vi "Prepare.vi"(8 "error in (no error)":errorcluster, 9 "Wavefom Sequence":T4, 10 "TDMS Name Mapping":T3, 11 "Resource Settings":T2={"FGEN Resource"="", "DAQmx Resource"="", "TDMS File Path"=path "", "Scope Resource"="", "Scope Config File Path"=path "", "Reference Position"=50.0} {"Reference Position" format="%#_g%"}) -> (0 "error out":errorcluster, 3 "Panel State Data Out":T1)   [LabVIEW 2025]
uses:
  Typedef/Test Panel State Data.ctl
  a73cb824-e8e3-43f7-ba20-95578727caf9.vi
  51479c3b-831f-4f08-87c6-485a7376d69e.vi
  Typedef/TDMS Name Mapping.ctl
  Typedef/Resource Settings.ctl
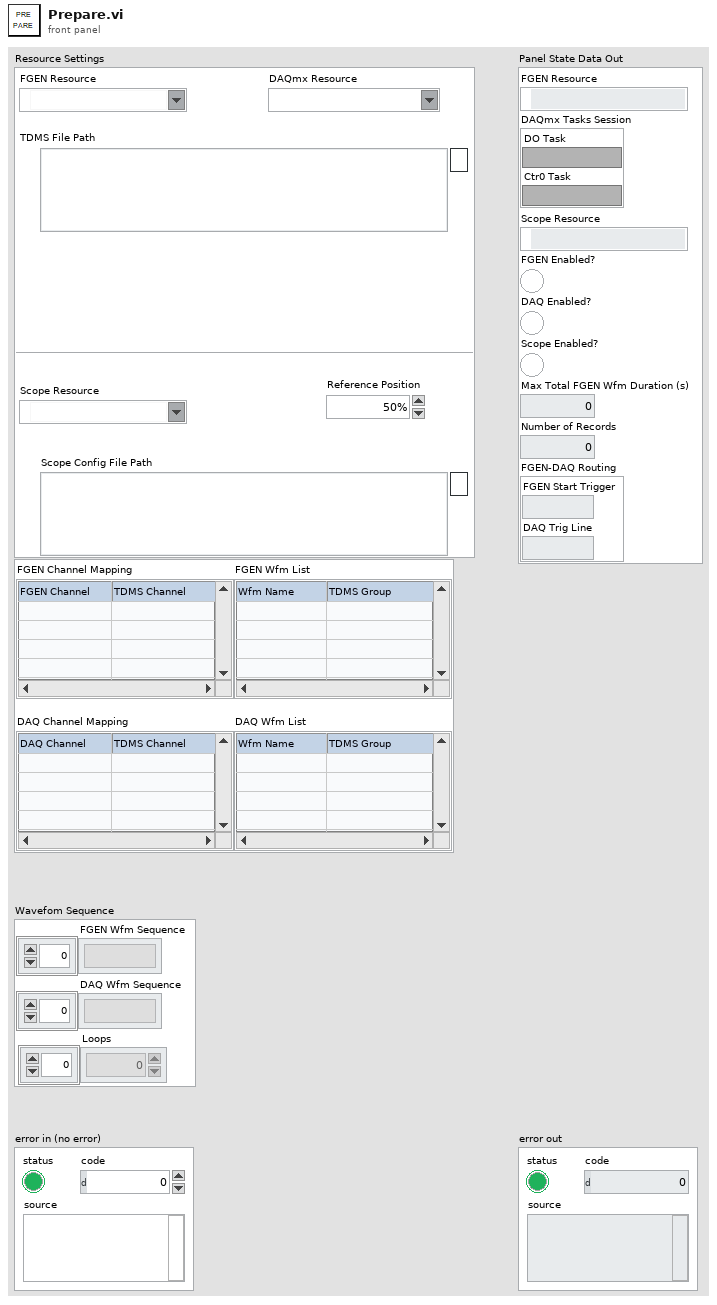
[diagram p1: front panel]
types:
  T1 = typedef "Test Panel State Data.ctl" = cluster{"FGEN Resource":refnum<k15>, "DAQmx Tasks Session":cluster{"DO Task":refnum<k21>, "Ctr0 Task":refnum<k21>}, "Scope Resource":refnum<k15>, "FGEN Enabled?":bool, "DAQ Enabled?":bool, "Scope Enabled?":bool, "Max Total FGEN Wfm Duration (s)":dbl, "Number of Records":i32, "FGEN-DAQ Routing":cluster{"FGEN Start Trigger":string, "DAQ Trig Line":string}}
  T2 = typedef "Resource Settings.ctl" = cluster{"FGEN Resource":refnum<k15>, "DAQmx Resource":tag, "TDMS File Path":path, "Scope Resource":refnum<k15>, "Scope Config File Path":path, "Reference Position":dbl}
  T3 = typedef "TDMS Name Mapping.ctl" = cluster{"FGEN Channel Mapping":string[][], "DAQ Channel Mapping":string[][], "FGEN Wfm List":string[][], "DAQ Wfm List":string[][]}
  T4 = cluster{"FGEN Wfm Sequence":string[], "DAQ Wfm Sequence":string[], "Loops":i32[]}
  T5 = cluster{"DAQ Channels":string[], "Sample Rate":dbl, "DAQ Wfm Map":map{string, digitalwaveform}, "DAQ Wfm Sequence":string[], "Loops":i32[]}
  T6 = cluster{"FGEN Channels":string[], "Sample Rate":dbl, "FGEN Wfm Map":map{string, waveform(dbl)[]}, "FGEN Wfm Sequence":string[], "Loops":i32[], "Gain Per Channel":dbl[]}
  T7 = cluster{"DO Task":refnum<k21>, "Ctr0 Task":refnum<k21>}
  T8 = cluster{"Scope Config File Path":path, "Reference Position":dbl, "Numeric":i32}
  T9 = cluster{"FGEN Start Trigger":string, "DAQ Trig Line":string}
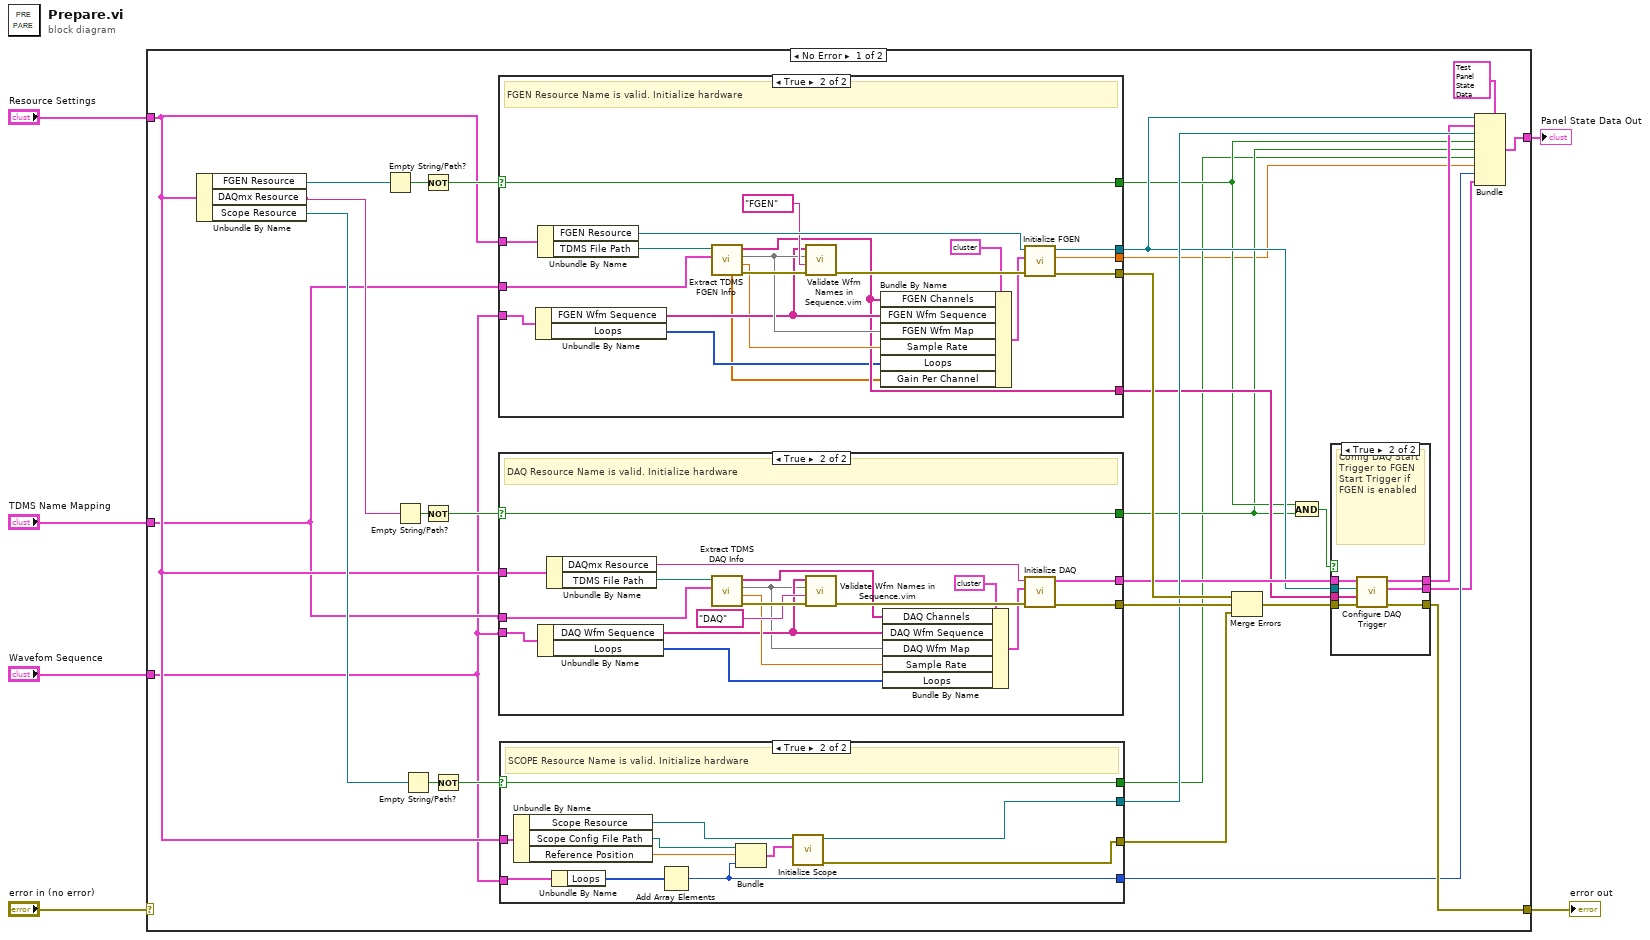
[diagram p0: block diagram]
diagram:
  n1 = case shown="No Error" "error in (no error)" {
    selector: "error in (no error)" -> [_ w99]
    tunnel: "Resource Settings" -> [w24 _]
    tunnel: "TDMS Name Mapping" -> [w21 _]
    tunnel: "Wavefom Sequence" -> [w20 _]
    tunnel: [w14 w99] -> w6
    tunnel: [w37 _] -> w1
    frame No Error {
      n2 = Unbundle By Name(w24) -> ("FGEN Resource"=w36:refnum<k15>, "DAQmx Resource"=w35:tag, "Scope Resource"=w34:refnum<k15>)
      n3 = Empty String/Path?(string/path=w36) -> (empty?=w33:bool)
      n4 = Empty String/Path?(string/path=w35) -> (empty?=w30:bool)
      n5 = Empty String/Path?(string/path=w34) -> (empty?=w26:bool)
      n6 = Not(x=w33) -> (.not. x?=w31:bool)
      n7 = Not(x=w30) -> (.not. x?=w29:bool)
      n8 = Not(x=w26) -> (.not. x?=w25:bool)
      n9 = case shown="True" w31 {
        selector: w31 -> [w78 w89]
        tunnel: w24 -> [_ w94]
        tunnel: w21 -> [_ w96]
        tunnel: w20 -> [_ w92]
        tunnel: [_ w90] -> w16
        tunnel: [w78 w89] -> w12
        tunnel: [_ w85] -> w27
        tunnel: [_ w84] -> w17
        tunnel: [_ w83] -> w9
        frame False {
          # "FGEN Resource Name is empty. Not initialized"
        }
        frame True {
          # "FGEN Resource Name is valid. Initialize hardware"
          n10 = Unbundle By Name(w92) -> ("FGEN Wfm Sequence"=w87:string[], "Loops"=w80:i32[])
          n11 = Unbundle By Name(w94) -> ("FGEN Resource"=w95:refnum<k15>, "TDMS File Path"=w97:path)
          n12 = call "Extract TDMS FGEN Info.vi"("TDMS Name Mapping"=w96, "TDMS File Path"=w97) -> ("error out"=w98:errorcluster, "FGEN Sample Rate"=w86:dbl, "FGEN Wfm Map"=w88:map{string, waveform(dbl)[]}, "FGEN Channels"=w84:string[], "Gain Per Channel"=w79:dbl[])  [unwired: 5 in]
          n13 = call "Validate Wfm Names in Sequence.vim"("error in"=w98, "Wfm Resource Type"="FGEN", "Wfm Map"=w88, "Wfm Sequence"=w87) -> ("error out"=w93:errorcluster)  [unwired: 6 in, 1 out]
          n14 = Bundle By Name(cluster=T6 {"FGEN Channels"=[], "Sample Rate"=0.0, "FGEN Wfm Map"={}, "FGEN Wfm Sequence"=[], "Loops"=[], "Gain Per Channel"=[]} ("FGEN Settings"), "FGEN Channels"=w84, "FGEN Wfm Sequence"=w87, "FGEN Wfm Map"=w88, "Sample Rate"=w86, "Loops"=w80, "Gain Per Channel"=w79) -> (w81:T6)
          n15 = call "Initialize FGEN.vi"("error in (no error)"=w93, "FGEN Settings"=w81, "FGEN Resource In"=w95) -> ("error out"=w85:errorcluster, "Total Wfm Duration (s)"=w83:dbl, "FGEN Resource Out"=w90:refnum<k15>)  [unwired: 6 in]
        }
      }
      n16 = case shown="True" w29 {
        selector: w29 -> [w59 w70]
        tunnel: w24 -> [_ w74]
        tunnel: w21 -> [_ w75]
        tunnel: w20 -> [_ w72]
        tunnel: [w59 w70] -> w11
        tunnel: [_ w64] -> w28
        tunnel: [_ w63] -> w18
        frame False {
          # "DAQ Resource Name is empty. Not initialized"
        }
        frame True {
          # "DAQ Resource Name is valid. Initialize hardware"
          n17 = Unbundle By Name(w72) -> ("DAQ Wfm Sequence"=w67:string[], "Loops"=w61:i32[])
          n18 = Unbundle By Name(w74) -> ("DAQmx Resource"=w66:tag, "TDMS File Path"=w76:path)
          n19 = call "Extract TDMS DAQ Info.vi"("TDMS Name Mapping"=w75, "TDMS File Path"=w76) -> ("error out"=w77:errorcluster, "DAQ Sample Rate"=w68:dbl, "DAQ Wfm Map"=w65:map{string, digitalwaveform}, "DAQ Channels"=w69:string[])  [unwired: 6 in]
          n20 = call "Validate Wfm Names in Sequence.vim"("error in"=w77, "Wfm Resource Type"="DAQ", "Wfm Map"=w65, "Wfm Sequence"=w67) -> ("error out"=w73:errorcluster)  [unwired: 6 in, 1 out]
          n21 = Bundle By Name(cluster=T5 {"DAQ Channels"=[], "Sample Rate"=0.0, "DAQ Wfm Map"={}, "DAQ Wfm Sequence"=[], "Loops"=[]} ("DAQ Settings"), "DAQ Channels"=w69, "DAQ Wfm Sequence"=w67, "DAQ Wfm Map"=w65, "Sample Rate"=w68, "Loops"=w61) -> (w60:T5)
          n22 = call "Initialize DAQ.vi"("error in (no error)"=w73, "DAQ Settings"=w60, "DAQmx Resource"=w66) -> ("error out"=w64:errorcluster, "DAQmx Tasks"=w63:T7)  [unwired: 7 in]
        }
      }
      n23 = case shown="True" w25 {
        selector: w25 -> [w47 w51]
        tunnel: w24 -> [_ w58]
        tunnel: [_ w56] -> w23
        tunnel: [_ w55] -> w22
        tunnel: w20 -> [_ w54]
        tunnel: [w47 w51] -> w10
        tunnel: [_ w50] -> w8
        frame False {
          # "SCOPE Resource Name is empty. Not initialized"
        }
        frame True {
          # "SCOPE Resource Name is valid. Initialize hardware"
          n24 = Unbundle By Name(w58) -> ("Scope Resource"=w57:refnum<k15>, "Scope Config File Path"=w52:path, "Reference Position"=w49:dbl)
          n25 = Unbundle By Name(w54) -> ("Loops"=w53:i32[])
          n26 = Add Array Elements(numeric array=w53) -> (sum=w50:i32)
          n27 = Bundle("Scope Config File Path"=w52, "Reference Position"=w49, "Numeric"=w50) -> (w48:T8)  [unwired: 1 in]
          n28 = call "Initialize Scope.vi"("Scope Settings"=w48, "Scope Resource"=w57) -> ("error out"=w55:errorcluster, "Scope Resource"=w56:refnum<k15>)  [unwired: 8 in]
        }
      }
      n29 = Merge Errors(w27, w28, w22) -> (w19:errorcluster)
      n30 = And(x=w12, y=w11) -> (x .and. y?=w13:bool)
      n31 = case shown="True" w13 {
        tunnel: w19 -> [w38 w46]
        tunnel: w18 -> [w39 w45]
        tunnel: w17 -> [_ w44]
        tunnel: w16 -> [_ w43]
        tunnel: [w39 w42] -> w15
        tunnel: [w38 w41] -> w14
        tunnel: [_ w40] -> w7
        frame False {
        }
        frame True {
          # "Config DAQ Start Trigger to FGEN Start Trigger if FGEN is enabled"
          n32 = call "Configure DAQ Trigger.vi"("error in (no error)"=w46, "FGEN Channels"=w44, "FGEN Resource"=w43, "DAQmx Tasks In"=w45) -> ("error out"=w41:errorcluster, "FGEN-DAQ Routing"=w40:T9, "DAQmx Tasks Out"=w42:T7)  [unwired: 5 in]
        }
      }
      n33 = Bundle(cluster=T1 {"FGEN Resource"="", "DAQmx Tasks Session"={"DO Task"="", "Ctr0 Task"=""}, "Scope Resource"="", "FGEN Enabled?"=FALSE, "DAQ Enabled?"=FALSE, "Scope Enabled?"=FALSE, "Max Total FGEN Wfm Duration (s)"=0.0, "Number of Records"=0, "FGEN-DAQ Routing"={"FGEN Start Trigger"="", "DAQ Trig Line"=""}} ("Panel State Data Out 2"), "FGEN Resource"=w16, "DAQmx Tasks Session"=w15, "Scope Resource"=w23, "FGEN Enabled?"=w12, "DAQ Enabled?"=w11, "Scope Enabled?"=w10, "Max Total FGEN Wfm Duration (s)"=w9, "Number of Records"=w8, "FGEN-DAQ Routing"=w7) -> (w37:T1)
    }
    frame Error {
    }
  }
  "error out" <- w6
  "Panel State Data Out" <- w1
